vi "PPMS.Set Get All.vi"(8 "error in (no error)":errorcluster, 10 "Data":variant, 11 "instrument.PPMS":refnum<class "instrument.PPMS.lvclass">) -> (0 "error out":errorcluster, 3 "instrument.PPMS out":refnum<class "instrument.PPMS.lvclass">)   [LabVIEW 2019]
uses:
  Typedefs/PPMS.Chamber Command--enum.ctl
  instrument.PPMS.lvclass
  9fd503d5-6126-44b4-9732-3eced29da0a7.vi
  <userlib>/LevyLab/Instrument Framework/Instrument Types/Cryostat/Typedefs/Set Chamber--cluster.ctl
  <userlib>/LevyLab/Instrument Framework/Instrument Types/Cryostat/Instrument.Cryostat.lvclass
  C:/Program Files (x86)/National Instruments/LabVIEW 2019/user.lib/LevyLab/Instrument Framework/Instrument Types/Cryostat/Instrument.Cryostat.lvclass
  C:/Program Files (x86)/National Instruments/LabVIEW 2019/user.lib/LevyLab/Instrument Framework/SMOs/Instrument/Instrument.lvclass
  C:/Program Files (x86)/National Instruments/LabVIEW 2019/vi.lib/JKI/JKI SMO/SMO/SMO.lvclass
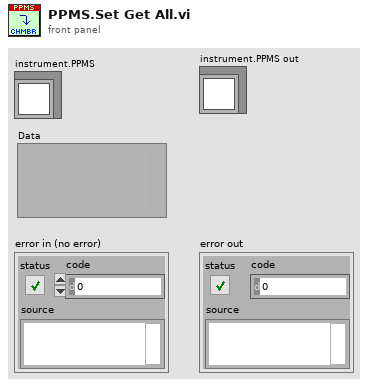
[diagram p1: front panel]
types:
  T1 = typedef "Instrument.Cryostat.lvclass/Set Chamber--cluster.ctl" = cluster{"Action":string}
  T2 = typedef "instrument.PPMS.lvclass/PPMS.Chamber Command--enum.ctl" = string
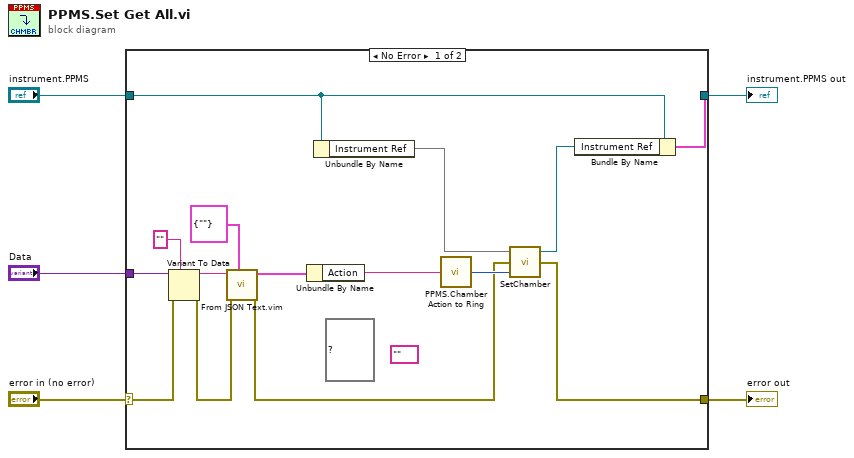
[diagram p0: block diagram]
diagram:
  n1 = case shown="No Error" "error in (no error)" {
    selector: "error in (no error)" -> [w13 w22]
    tunnel: [w19 w22] -> w5
    tunnel: "instrument.PPMS" -> [w10 w21]
    tunnel: [w11 w21] -> w2
    tunnel: "Data" -> [w14 _]
    frame No Error {
      (unwired) map{u16, string} {0="Seal", 1="PurgeAndSeal", 2="VentAndSeal", 3="PumpContinuous", 4="VentContinuous", 5="HighVacuum"} ("Map")
      (unwired) T2 "" ("Code")
      n2 = Variant To Data(error in=w13, type="", Variant=w14) -> (data=w16:string, error out=w15:errorcluster)
      n3 = call "From JSON Text.vim"("Data Type and Default Value"=T1 {"Action"=""} ("Set Chamber"), "error in (no error)"=w15, "JSON"=w16) -> ("error out"=w12:errorcluster, "Data out"=w7:T1)  [unwired: 7 in]
      n4 = Unbundle By Name(w7) -> ("Action"=w6:string)
      n5 = Unbundle By Name(w10) -> ("Instrument Ref"=w20)
      n6 = call "PPMS.Chamber Action to Ring.vi"("Data in"=w6) -> ("Value"=w18:u16)
      n7 = call "SetChamber.vi"("Code"=w18, "error in (no error)"=w12, "Instrument Ref In"=w20) -> ("error out"=w19:errorcluster, "Instrument Ref Out"=w9:refnum<k24>)  [unwired: 1 out]
      n8 = Bundle By Name(cluster=w10, "Instrument Ref"=w9) -> (w11:cluster{})
    }
    frame Error {
    }
  }
  "error out" <- w5
  "instrument.PPMS out" <- w2
